vi "Naughty VI Test.vi"   [LabVIEW 2024]
uses:
  297d9782-6bef-44c7-b1e5-d0cf554b8d0d.vi
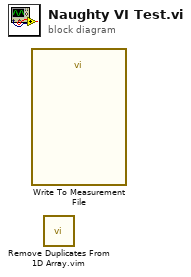
[diagram p0: block diagram]
diagram:
  n1 = call "Write To Measurement File"() -> ()  [unwired: 17 in, 3 out]
  n2 = call "Remove Duplicates From 1D Array.vim"() -> ()  [unwired: 11 in, 1 out]
